vi "_unittest Add Test Group.vi"(8 "error in (no error)":errorcluster, 11 "Test Group":string) -> (0 "error out":errorcluster)   [LabVIEW 2018, in "labview_json_tests.lvlib"]
uses:
  labview_json_tests.lvlib
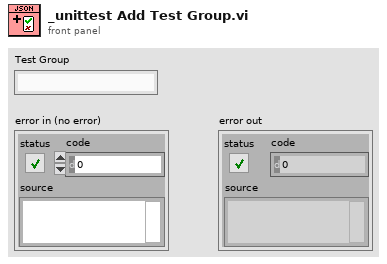
[diagram p1: front panel]
types:
  T1 = enum8{"Report", "Add Test Group", "Add Test Case"}
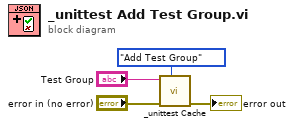
[diagram p0: block diagram]
diagram:
  n1 = call "_unittest Cache.vi"("Action"=T1."Add Test Group", "error in (no error)"="error in (no error)", "Test Name"="Test Group") -> ("error out"=→"error out":errorcluster)  [unwired: 7 in, 1 out]
